vi "Configure osciloscopio FULL con generador.vi"(0 "Visa MDO3104":refnum<visa-resource-name>="USB0::0x0699::0x0408::C016316::INSTR", 5 "Amplitud":dbl, 11 "error out":errorcluster, 12 "Esperar a completar estadisticas":bool, 13 "Configurar Osciloscopio":bool=TRUE) -> (4 "VISA resource name out 2":refnum<visa-resource-name>="Osciloscopio_Tek_MDO3104", 6 "Array":dbl[](array[numeric])=[0.4730278, 0.4040874, 0.8764885, 3.0701e-09], 8 "Ch1+Ch2":dbl=0.8771152, 10 "Math (CH1-CH2)":dbl=0.8764885, 15 "error out 2":errorcluster)   [LabVIEW 2019]
doc: "Atencion!!!!\nEl osciloscopio algunas veces no consigue medir correctamente la funcion matematica dando valores de tension por debajo del que muestra la pantalla y un ancho de pulso de infinito.\nPor ello hay dos salidas Ch1+Ch2 que seria la suma de las medias de las amplitudes de ambos canales o bien Math (ch1-ch2) que seria la media de las resta punto a punto de los dos canales.\nGustavo piensa que es mejor MATH yo creo que es mejor la otra ya veremos como la cableo."
uses:
  Tektronix DPO MSO 2000 4000 Series/Tektronix DPO MSO 2000 4000 Series.lvlib
panel:
  in  "Tolerance":dbl=10.0 format="%#_g%%"
  in  "V Theorical":dbl=1.0096
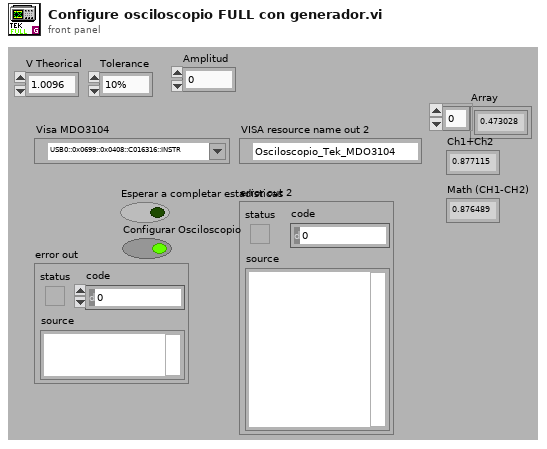
[diagram p1: front panel]
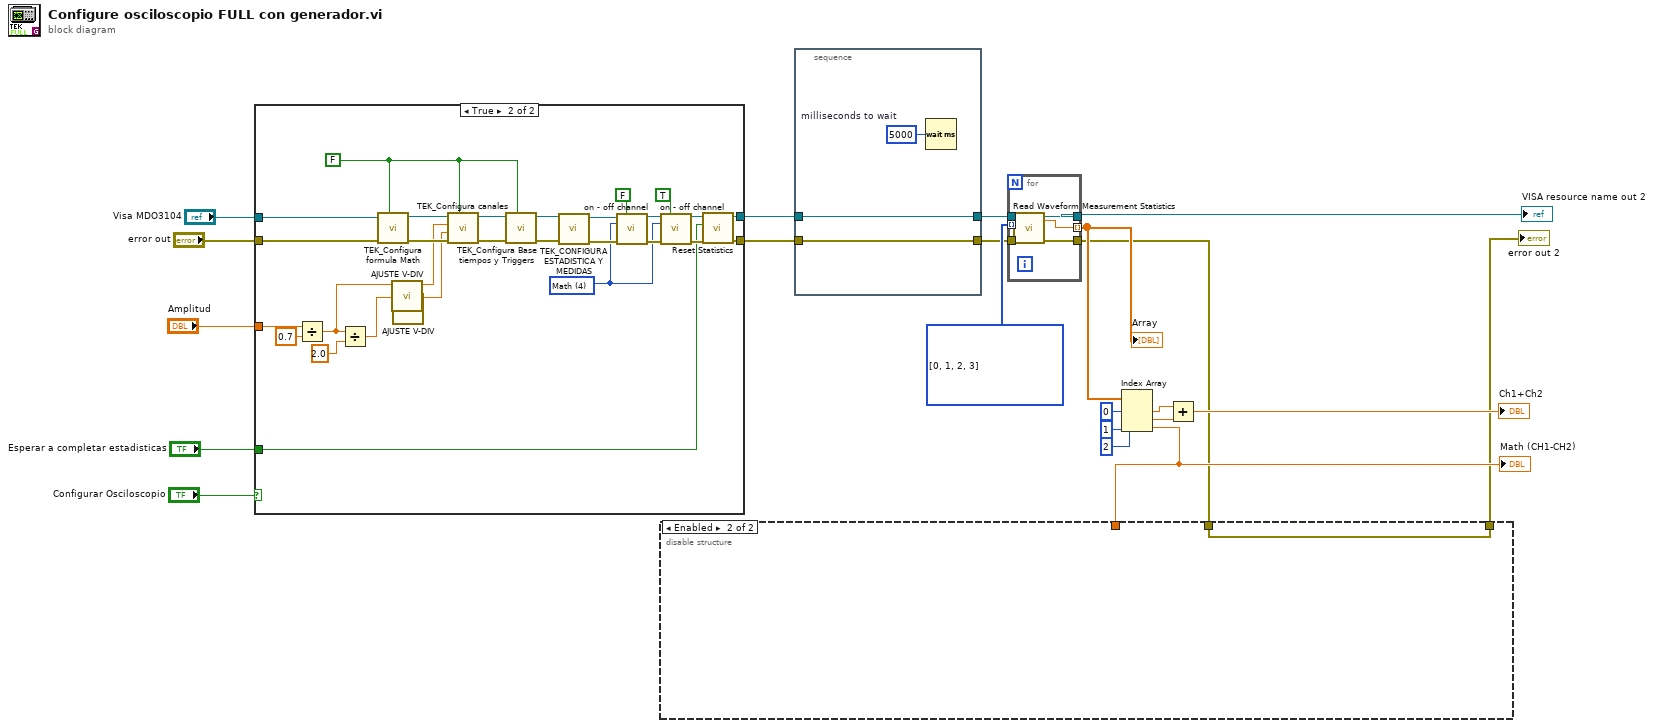
[diagram p0: block diagram]
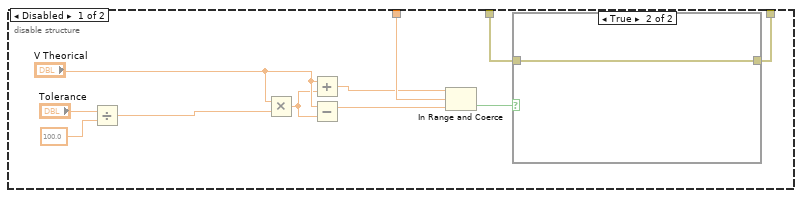
[diagram p2: hidden frame]
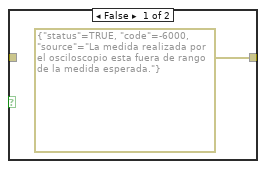
[diagram p3: hidden frame]
diagram:
  w19 = i32[] [0, 1, 2, 3] items=["Measurement 1", "Measurement 2", "Measurement 3", "Measurement 4"]
  n1 = case shown="True" "Configurar Osciloscopio" {
    tunnel: "error out" -> [w22 w50]
    tunnel: "Visa MDO3104" -> [w23 w49]
    tunnel: [w22 w42] -> w2
    tunnel: [w23 w41] -> w4
    tunnel: "Esperar a completar estadisticas" -> [_ w31]
    tunnel: "Amplitud" -> [_ w24]
    frame False {
    }
    frame True {
      w32 = u16 4 items=["Channel 1", "Channel 2", "Channel 3", "Channel 4", "Math", "Reference 1", "Reference 2", "Reference 3", "Reference 4", "Bus 1", "Bus 2"] ("Channel (0: Channel 1)")
      w51 = FALSE ("Debug")
      n2 = Divide(x=w24, y=0.7) -> (x/y=w28:dbl)
      n3 = Divide(x=w28, y=2.0) -> (x/y=w26:dbl)
      n4 = call "TEK_Configura formula Math.vi"("Debug"=w51, "error out"=w50, "VISA resource name out 2"=w49) -> ("error out 2"=w45:errorcluster, "VISA resource name out"=w46:refnum<visa-resource-name>)  [unwired: 7 in]
      n5 = call "AJUSTE V-DIV.vi"("y 2"=w28) -> ("y"=w27:dbl)  [unwired: 10 in]
      n6 = call "AJUSTE V-DIV.vi"("y 2"=w26) -> ("y"=w25:dbl)  [unwired: 10 in]
      n7 = call "TEK_Configura canales.vi"("Debug"=w51, "error out 2"=w45, "ch2 ch3 V/Div"=w25, "Math V/Div"=w27, "VISA resource name out"=w46) -> ("error out"=w48:errorcluster, "VISA resource name out 2"=w47:refnum<visa-resource-name>)  [unwired: 5 in]
      n8 = call "TEK_Configura Base tiempos y Triggers.vi"("Debug"=w51, "error out 2"=w48, "VISA resource name out 2"=w47) -> ("error out"=w43:errorcluster, "VISA resource name out"=w44:refnum<visa-resource-name>)  [unwired: 7 in]
      n9 = call "TEK_CONFIGURA ESTADISTICA Y MEDIDAS.vi"("error out"=w43, "VISA resource name out"=w44) -> ("error out 2"=w33:errorcluster, "VISA resource name out 2"=w34:refnum<visa-resource-name>)  [unwired: 8 in]
      n10 = call "on - off channel.vi"("VISA resource name"=w34, "Enable Channel (T: Enable)"=FALSE, "Channel (0: Channel 1)"=w32, "error in (no error)"=w33) -> ("VISA resource name out"=w40:refnum<visa-resource-name>, "error out"=w39:errorcluster)  [unwired: 10 in]
      n11 = call "on - off channel.vi"("VISA resource name"=w40, "Enable Channel (T: Enable)"=TRUE, "Channel (0: Channel 1)"=w32, "error in (no error)"=w39) -> ("VISA resource name out"=w37:refnum<visa-resource-name>, "error out"=w38:errorcluster)  [unwired: 10 in]
      n12 = call "Reset Statistics.vi"("error in (no error)"=w38, "Wait medida"=w31, "VISA resource name"=w37) -> ("error out"=w42:errorcluster, "VISA resource name out"=w41:refnum<visa-resource-name>)  [unwired: 7 in]
    }
  }
  n13 = stacked-sequence {
    tunnel: w4 -> [w54]
    tunnel: [w54] -> w3
    tunnel: w2 -> [w53]
    tunnel: [w53] -> w1
    frame #0 {
      w52 = u32 5000  # milliseconds to wait
      n14 = Wait (ms)(milliseconds to wait=w52) -> ()  [unwired: 1 out]
    }
  }
  n15 = for {
    tunnel: [w60] -> w9
    tunnel: [w59] -> w18
    tunnel: [w58] -> w17 mode=indexing
    tunnel: w1 -> [w57]
    tunnel: w3 -> [w56]
    tunnel: w19 -> [w55] mode=indexing
    n16 = call "Read Waveform Measurement Statistics.vi"("error in (no error)"=w57, "Measurement Number (0: Measurement 1)"=w55, "VISA resource name"=w56) -> ("error out"=w60:errorcluster, "VISA resource name out"=w59:refnum<visa-resource-name>, "Mean Value"=w58:dbl)  [unwired: 3 in, 3 out]
  }
  "VISA resource name out 2" <- w18
  "Array" <- w17
  n17 = Index Array(array=w17, index #1=0 ("index"), index #2=1 ("index"), index #3=2 ("index")) -> (element #1=w13:dbl, element #2=w12:dbl, element #3=w10:dbl)
  "Math (CH1-CH2)" <- w10
  n18 = disable-structure shown="Enabled" {
    disable-tunnel: w10 -> [w71 _]
    disable-tunnel: w9 -> [w62 w74]
    disable-tunnel: [w61 w74] -> w8
    frame Disabled {
      n19 = Divide(x="Tolerance", y=100.0) -> (x/y=w64:dbl)
      n20 = Multiply(x="V Theorical", y=w64) -> (x*y=w69:dbl)
      n21 = Add(x="V Theorical", y=w69) -> (x+y=w68:dbl)
      n22 = Subtract(x="V Theorical", y=w69) -> (x-y=w67:dbl)
      n23 = In Range and Coerce(upper limit=w68, x=w71, lower limit=w67) -> (In Range?=w63:bool)  [unwired: 1 out]
      n24 = case shown="True" w63 {
        tunnel: w62 -> [_ w73]
        tunnel: [errorcluster {"status"=TRUE, "code"=-6000, "source"="La medida realizada por el osciloscopio esta fuera de rango de la medida esperada."} ("error out") w73] -> w61
        frame False {
        }
        frame True {
        }
      }
    }
    frame Enabled {
    }
  }
  "error out 2" <- w8
  n25 = Add(x=w13, y=w12) -> (x+y=→"Ch1+Ch2":dbl)
